vi "KM_get_sweep V1.vi.vi"(6 "N":i32=100, 8 "Error In":errorcluster, 9 "omega0 (Hz)":dbl=44500.0, 10 "gamma (Hz)":dbl=1000.0, 11 "Address":string="DEV3523") -> (0 "Error Out":errorcluster, 1 "freq out (Hz)":dbl[](array[numeric]), 2 "voltage out (V)":cdb[](array[numeric]))   [LabVIEW 2016]
uses:
  array - generate range.vi
  <instrlib>/Zurich Instruments LabOne/Zurich Instruments LabOne.lvlib
panel:
  in  "timeconstant (s)":dbl=1.0 format="%#_13g"
  out "Selected Device":string="DEV3523"
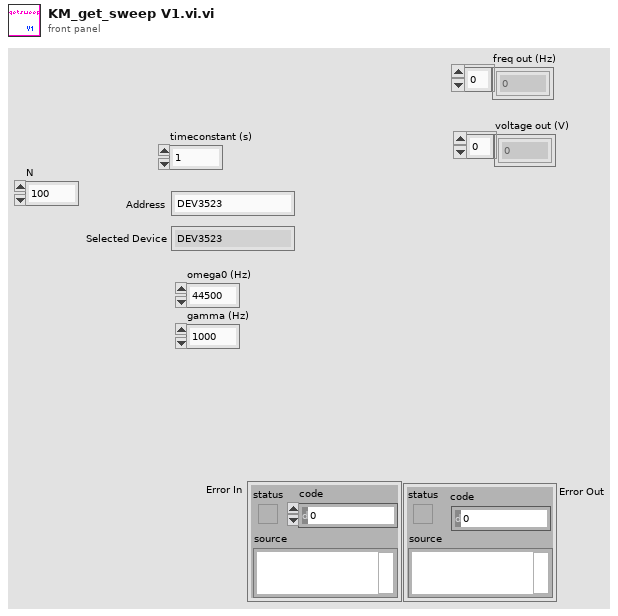
[diagram p1: front panel]
types:
  T1 = typedef "Zurich Instruments LabOne.lvlib/ziTypeHandle.ctl" = cluster{"handleValid":bool, "Conn":u64, "Path Prefix":string, "Handle":u64, "Connected":bool, "Clockbase(s)":dbl}
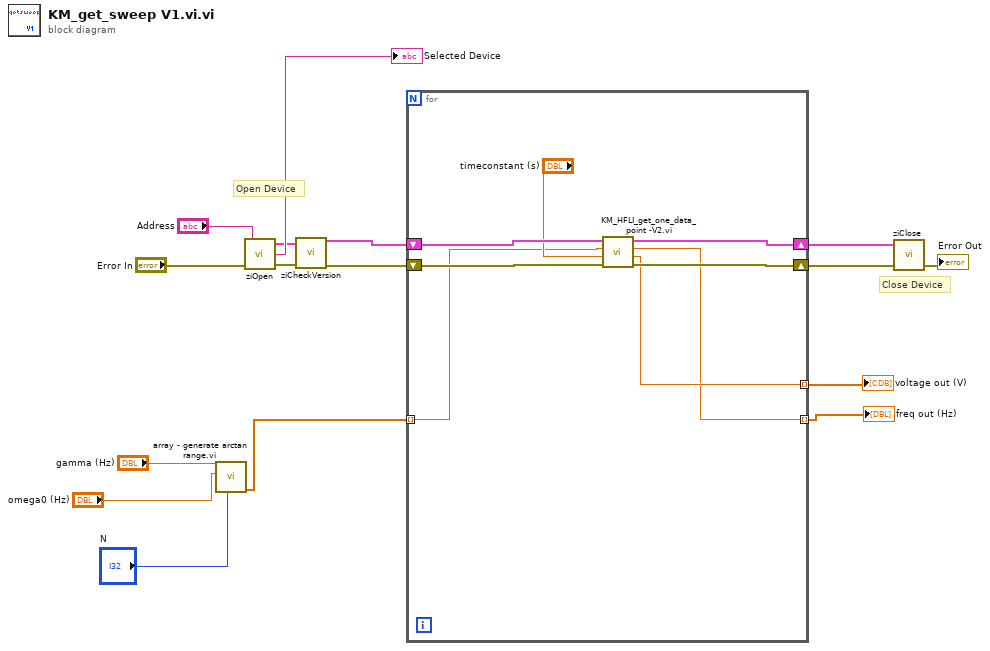
[diagram p0: block diagram]
diagram:
  # "Close Device"
  # "Open Device"
  n1 = call "array - generate arctan range.vi.vi"("N"="N", "omega0"="omega0 (Hz)", "gamma"="gamma (Hz)") -> ("Array"=w5:dbl[])  [unwired: 8 in]
  n2 = call "ziOpen.vi"("Error In"="Error In", "Address"="Address") -> ("Error Out"=w12:errorcluster, "Selected Device"=→"Selected Device":string, "HandleOut"=w13:T1)  [unwired: 2 out]
  n3 = call <instrlib>:"ziCheckVersion.vi"("Handle In"=w13, "Error In"=w12) -> ("Handle Out"=w11:T1, "Error Out"=w10:errorcluster)  [unwired: 12 in]
  n4 = for {
    shift-right: [w21] -> w8
    shift-left: w11 -> [w24]
    shift-right: [w22] -> w9
    shift-left: w10 -> [w23]
    tunnel: w5 -> [w19] mode=indexing
    tunnel: [w17] -> w1 mode=indexing
    tunnel: [w18] -> w6 mode=indexing
    n5 = call "KM_HFLI_get_one_data_point -V2.vi.vi"("Error In"=w23, "timeconstant (s)"="timeconstant (s)", "Freq in (Hz)"=w19, "Handle In"=w24) -> ("Error Out"=w22:errorcluster, "z out (V)"=w18:cdb, "Freq out (Hz)"=w17:dbl, "Handle Out"=w21:T1)  [unwired: 4 in]
  }
  "voltage out (V)" <- w6
  "freq out (Hz)" <- w1
  n6 = call "ziClose.vi"("Error In"=w9, "Handle In"=w8) -> ("Error Out"=→"Error Out":errorcluster)  [unwired: 2 in, 1 out]
